vi "Create_Pos_array.vi"(2 "Traverse line":T1 {"Carrier_2 Q (l/min)" format="%#.2f"; "Row Duration (mins)" format="%#.1f"; "Row No" min=0; "Trace Gas Concentration (%)" min=0.0 format="%#_4f"; "Carrier_1 Q (l/min)" format="%#.4f"; "Start X" format="%#.2f"; "Start Y" format="%#.2f"; "Start Z" format="%#.2f"; "End X" format="%#.2f"; "End Y" format="%#.2f"; "End Z" format="%#.2f"; "Tunnel Speed" format="%#.2f"; "Averaging time (mins)" min=0.0 format="%#.2f"}) -> (5 "Traverse line Out":T1 {"Carrier_2 Q (l/min)" format="%#.2f"; "Row Duration (mins)" format="%#.1f"; "Row No" min=0; "Trace Gas Concentration (%)" min=0.0 format="%#_4f"; "Carrier_1 Q (l/min)" format="%#.4f"; "Start X" format="%#.2f"; "Start Y" format="%#.2f"; "Start Z" format="%#.2f"; "End X" format="%#.2f"; "End Y" format="%#.2f"; "End Z" format="%#.2f"; "Tunnel Speed" format="%#.2f"; "Averaging time (mins)" min=0.0 format="%#.2f"}, 6 "Error Messages":string, 7 "Array of Positions":sgl[][](array[numeric]) format="%.2f", 9 "Axis Traversed":enum16{"X traverse", "Y traverse", "Z traverse"}(ring))   [LabVIEW 2020]
uses:
  Traverse_cluster.ctl
  Spacing.ctl
  Controls/Multi_run_mode.ctl
  Globals/Extra_Commands_Global.vi
panel:
  # "X           Y          Z"
  # "Start"
  # "End"
  # "X           Y          Z"
  # "Start"
  # "End"
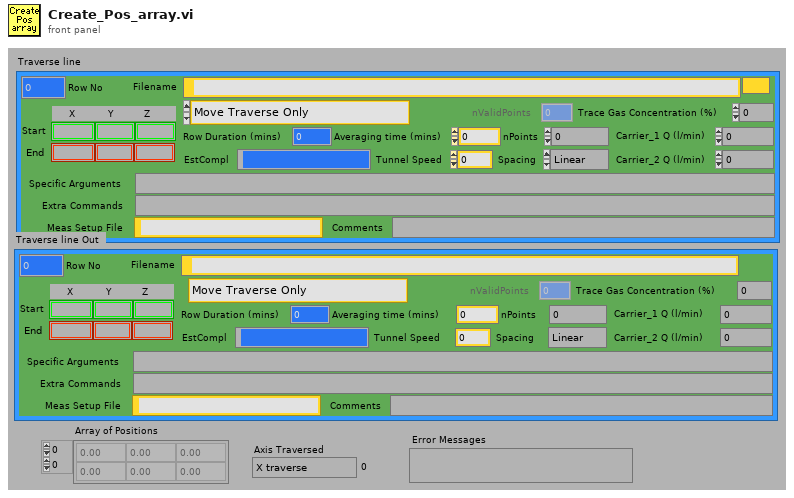
[diagram p1: front panel]
types:
  T1 = typedef "Traverse_cluster.ctl" = cluster{"Start X":sgl, "Start Y":sgl, "Start Z":sgl, "End X":sgl, "End Y":sgl, "End Z":sgl, "nPoints":i32, "Spacing":T2, "Filename":path, "Tunnel Speed":dbl, "Averaging time (mins)":dbl, "Extra Commands":string, "Carrier_1 Q (l/min)":dbl, "Carrier_2 Q (l/min)":dbl, "Trace Gas Concentration (%)":dbl, "Specific Arguments":string, "Comments":string, "Row No":i32, "Row Type Selector":T3, "EstCompl":string, "Row Duration (mins)":dbl, "nValidPoints":i32, "Meas Setup File":string}
  T2 = typedef "Spacing.ctl" = enum16{"Linear", "Log", "Gauss", "Specified", "N/A"}
  T3 = typedef "Multi_run_mode.ctl" = enum16{"Move Traverse Only", "Set Tunnel Speed Only", "Set Source Only", "Set Measurement Conditions", "Single Measurement", "Vertical Profile", "Lateral Profile", "Longitudinal Profile", "Multi-Axis Profile", "Explore Volume", "Auto Calibrate", "Meas Fast FID Bkgnd", "Check Beam Power", "Scanning Valve Measurement", "Run VI Named:", "Set ADAM Ch", "Wait (minutes)", "Send Message", "Synchronize With:", "Fall Back to this Row", "Turn Off Row Repeating", "Traverse 3D Volume", "Blank Row", "Jump to Fall Back Row"}
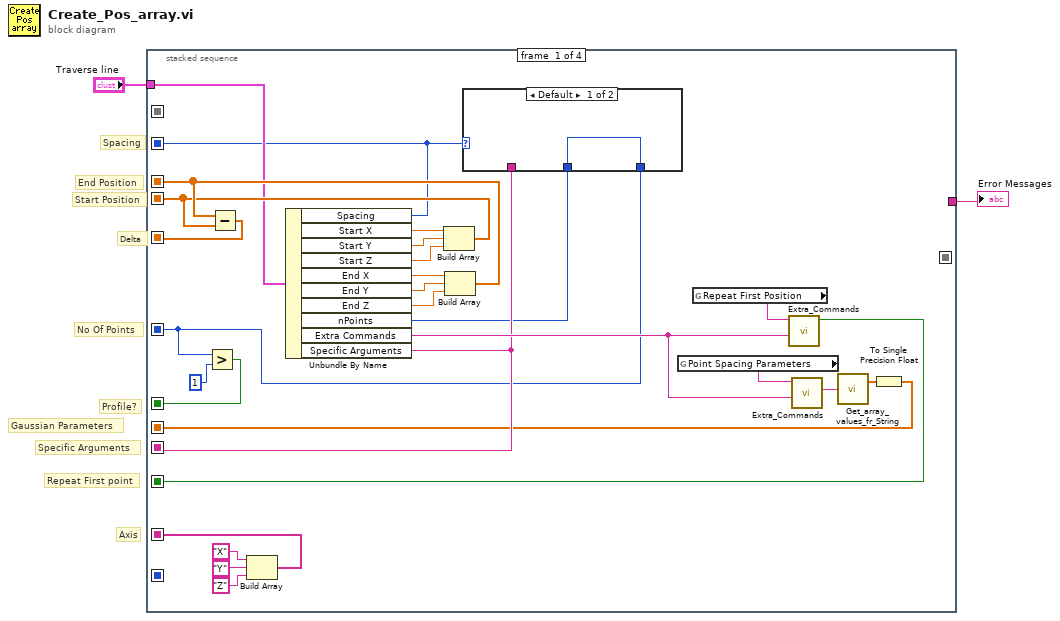
[diagram p0: block diagram]
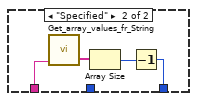
[diagram p2: hidden frame]
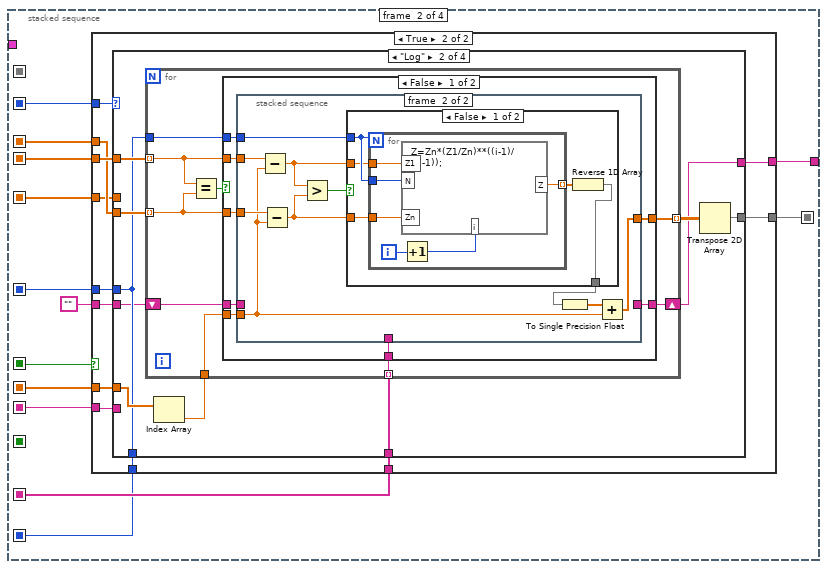
[diagram p3: hidden frame]
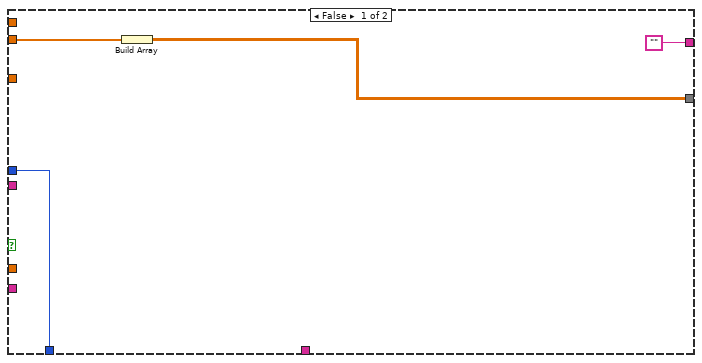
[diagram p4: hidden frame]
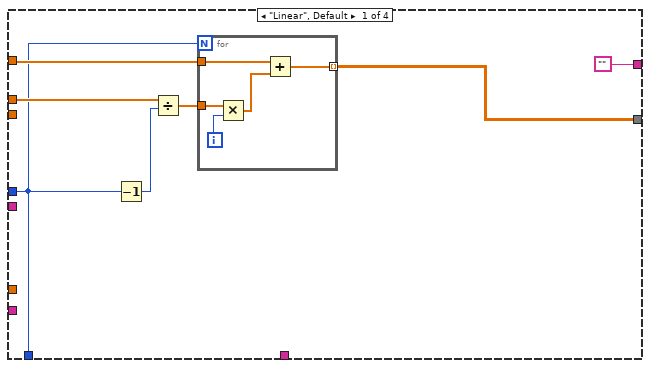
[diagram p5: hidden frame]
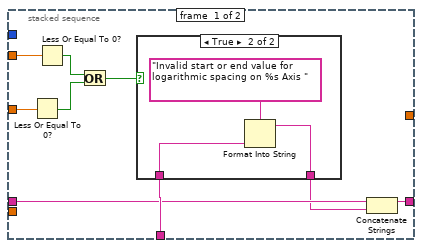
[diagram p6: hidden frame]
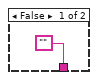
[diagram p7: hidden frame]
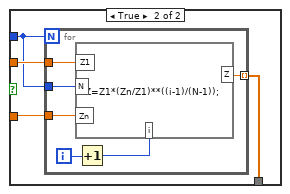
[diagram p8: hidden frame]
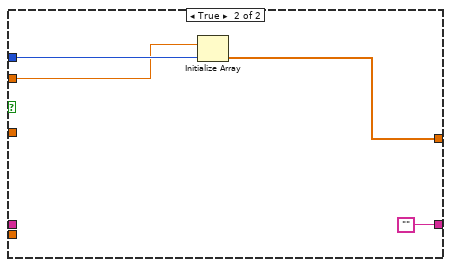
[diagram p9: hidden frame]
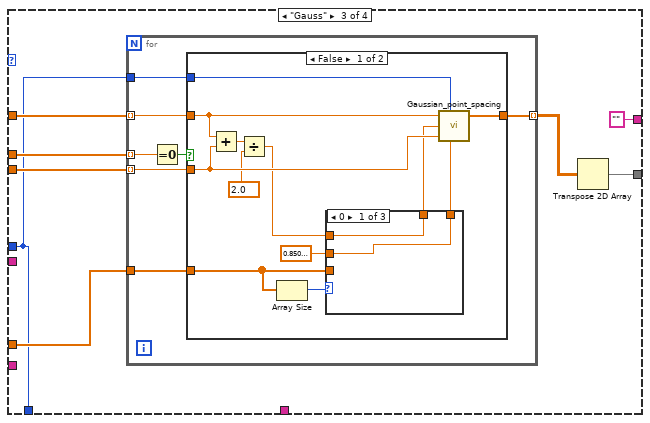
[diagram p10: hidden frame]
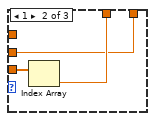
[diagram p11: hidden frame]
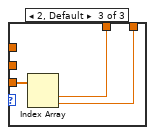
[diagram p12: hidden frame]
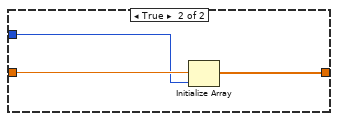
[diagram p13: hidden frame]
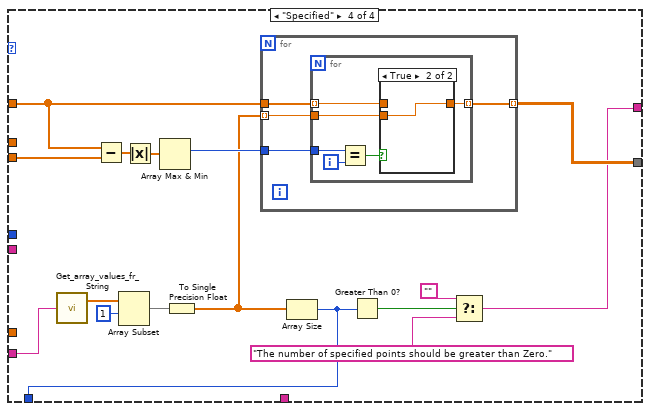
[diagram p14: hidden frame]
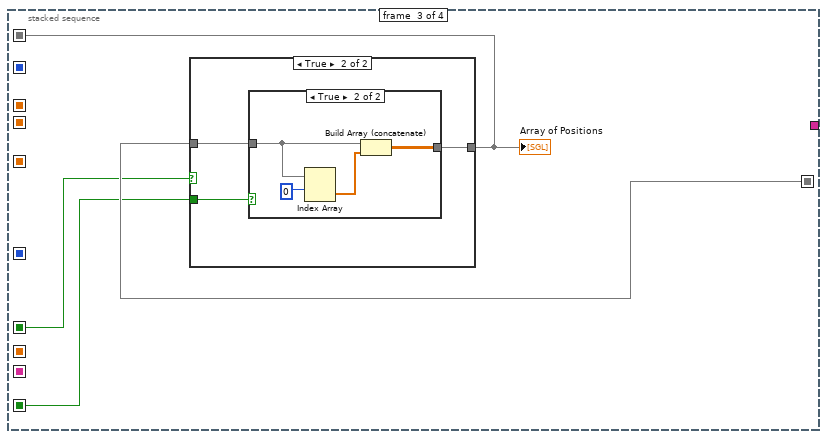
[diagram p16: hidden frame]
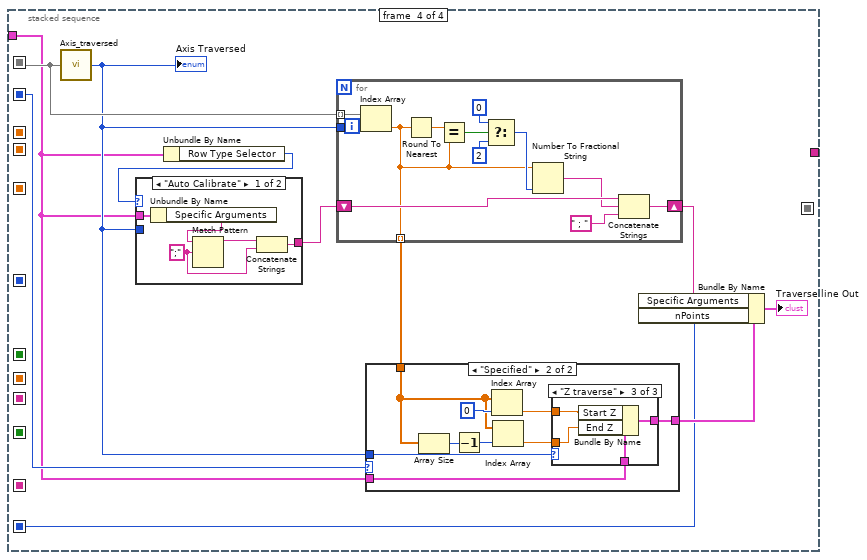
[diagram p19: hidden frame]
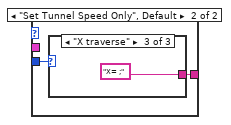
[diagram p20: hidden frame]
diagram:
  # "Gaussian Parameters"
  # "Axis"
  # "Profile?"
  # "Delta"
  # "Repeat First point"
  # "Spacing"
  # "No Of Points"
  # "Specific Arguments"
  # "End Position"
  # "Start Position"
  n1 = stacked-sequence {
    seq-local: [_ w47 _ _] -> [_ _ w220 _]
    seq-local: [w19 _ _ _] -> [_ w44 _ _]
    seq-local: [w22 _ _ _] -> [_ w42 _ _]
    seq-local: [w23 _ _ _] -> [_ w43 _ _]
    seq-local: [w6 _ _ _] -> [_ w40 _ _]
    seq-local: [w7 _ _ _] -> [_ w46 _ _]
    seq-local: [w8 _ _ _] -> [_ w45 _ w236]
    seq-local: [w13 _ _ _] -> [_ _ w219 _]
    seq-local: [w20 _ _ _] -> [_ w39 w218 _]
    seq-local: [w15 _ _ _] -> [_ w38 _ _]
    seq-local: [_ _ w217 _] -> [_ _ _ w240]
    seq-local: [w3 _ _ _] -> [_ w37 _ _]
    seq-local: [_ w36 _ _] -> [_ _ _ w230]
    tunnel: [_ w41 _ _] -> w2
    tunnel: "Traverse line" -> [w12 _ _ w231]
    frame #0 {
      n2 = Build Array("X", "Y", "Z") -> (w15:string[])
      n3 = Unbundle By Name(w12) -> ("Spacing"=w8:T2, "Start X"=w29:sgl, "Start Y"=w28:sgl, "Start Z"=w27:sgl, "End X"=w26:sgl, "End Y"=w25:sgl, "End Z"=w24:sgl, "nPoints"=w5:i32, "Extra Commands"=w10:string, "Specific Arguments"=w7:string)
      n4 = Build Array(w29, w28, w27) -> (w19:sgl[])
      n5 = Build Array(w26, w25, w24) -> (w23:sgl[])
      n6 = Subtract(x=w23, y=w19) -> (x-y=w22:sgl[])
      n7 = case shown="Default" w8 {
        tunnel: w7 -> [_ w34]
        tunnel: [w30 w31] -> w6
        tunnel: w5 -> [w30 _]
        frame Default {
        }
        frame "Specified" {
          n8 = call "Get_array_values_fr_String.vi"("String Value"=w34) -> ("String array"=w33:string[])  [unwired: 1 out]
          n9 = Array Size(array=w33) -> (size(s)=w32:i32)
          n10 = Decrement(x=w32) -> (x-1=w31:i32)
        }
      }
      n11 = Greater?(x=w6, y=1) -> (0:w20:bool)
      n12 = global read "Extra_Commands_Global.vi" "Point Spacing Parameters"() -> (w11:string)
      n13 = global read "Extra_Commands_Global.vi" "Repeat First Position"() -> (w14:string)
      n14 = call "Extra_Commands.vi"("String to Search"=w10, "Command"=w14) -> ("Command Found"=w13:bool)  [unwired: 1 in, 4 out]
      n15 = call "Extra_Commands.vi"("String to Search"=w10, "Command"=w11) -> ("String Value"=w9:string)  [unwired: 1 in, 4 out]
      n16 = call "Get_array_values_fr_String.vi"("String Value"=w9) -> ("Numeric Array"=w4:dbl[])  [unwired: 1 out]
      n17 = To Single Precision Float(number=w4) -> (single precision float=w3:sgl[])
    }
    frame #1 {
      n18 = case shown="True" w39 {
        tunnel: [w50 w63] -> w47
        tunnel: w46 -> [_ w62]
        tunnel: w45 -> [_ w61]
        tunnel: w44 -> [w51 w60]
        tunnel: w43 -> [_ w59]
        tunnel: w42 -> [_ w58]
        tunnel: w40 -> [w48 w57]
        tunnel: ["" w56] -> w41
        tunnel: w38 -> [_ w55]
        tunnel: w37 -> [_ w54]
        tunnel: [w48 w53] -> w36
        tunnel: "" -> [_ w52]
        frame False {
          n19 = Build Array(w51) -> (w50:sgl[][])
        }
        frame True {
          n20 = case shown="\"Log\"" w61 {
            tunnel: w59 -> [_ w84 w156 w199]
            tunnel: w60 -> [w69 w85 w157 w195]
            tunnel: w57 -> [w64 w77 w151 _]
            tunnel: [w70 w83 w155 w203] -> w63
            tunnel: w58 -> [w68 _ w158 _]
            tunnel: w62 -> [_ _ _ w204]
            tunnel: ["" w80 "" ("f") w200] -> w56
            tunnel: w55 -> [_ w81 _ _]
            tunnel: w54 -> [_ w79 w152 _]
            tunnel: [w64 w77 w151 w192] -> w53
            tunnel: w52 -> [_ w76 _ _]
            frame "Linear", Default {
              n21 = Decrement(x=w64) -> (x-1=w66:i32)
              n22 = Divide(x=w68, y=w66) -> (x/y=w67:sgl[])
              n23 = for {
                N: w64 -> [_]
                tunnel: w67 -> [w74]
                tunnel: w69 -> [w72]
                tunnel: [w71] -> w70 mode=indexing
                i -> [w75]
                n24 = Multiply(x=w74, y=w75) -> (x*y=w73:sgl[])
                n25 = Add(x=w72, y=w73) -> (x+y=w71:sgl[])
              }
            }
            frame "Log" {
              n26 = Index Array(array=w79) -> (element=w78:sgl)  [unwired: 1 in]
              n27 = for {
                tunnel: [w94] -> w82 mode=indexing
                tunnel: w85 -> [w87] mode=indexing
                tunnel: w84 -> [w86] mode=indexing
                tunnel: w77 -> [w93]
                tunnel: w81 -> [w91] mode=indexing
                shift-right: [w89] -> w80
                shift-left: w76 -> [w90]
                tunnel: w78 -> [w88]
                n28 = Equal?(x=w87, y=w86) -> (x = y?=w92:bool)
                n29 = case shown="False" w92 {
                  tunnel: w93 -> [w102 w149]
                  tunnel: w86 -> [w101 _]
                  tunnel: w87 -> [w100 w148]
                  tunnel: [w99 w150] -> w94
                  tunnel: w91 -> [w98 _]
                  tunnel: w90 -> [w97 _]
                  tunnel: [w96 ""] -> w89
                  tunnel: w88 -> [w95 _]
                  frame False {
                    n30 = stacked-sequence {
                      tunnel: [_ w123] -> w99
                      tunnel: w100 -> [w111 w122]
                      tunnel: w101 -> [w110 w121]
                      tunnel: w102 -> [_ w124]
                      tunnel: w98 -> [w106 _]
                      tunnel: w97 -> [w105 _]
                      tunnel: [w103 _] -> w96
                      tunnel: w95 -> [_ w120]
                      frame #0 {
                        n31 = Less Or Equal To 0?(x=w110) -> (x <= 0?=w109:bool)
                        n32 = Less Or Equal To 0?(x=w111) -> (x <= 0?=w108:bool)
                        n33 = Or(x=w108, y=w109) -> (x .or. y?=w107:bool)
                        n34 = case shown="True" w107 {
                          tunnel: w106 -> [_ w115]
                          tunnel: ["" w113] -> w104
                          frame False {
                          }
                          frame True {
                            n35 = Format Into String(format string="Invalid start or end value for logarithmic spacing on %s Axis " ("Format String"), w115) -> (resulting string=w113:string)  [unwired: 2 in, 1 out]
                          }
                        }
                        n36 = Concatenate Strings(w105, w104) -> (w103:string)
                      }
                      frame #1 {
                        n37 = Subtract(x=w122, y=w120) -> (x-y=w118:sgl)
                        n38 = Subtract(x=w121, y=w120) -> (x-y=w119:sgl)
                        n39 = Greater?(x=w118, y=w119) -> (0:w125:bool)
                        n40 = case shown="False" w125 {
                          tunnel: [w127 w137] -> w117
                          tunnel: w118 -> [w126 w140]
                          tunnel: w119 -> [w130 w139]
                          tunnel: w124 -> [w129 w138]
                          frame False {
                            n41 = for {
                              N: w129 -> [_]
                              tunnel: w130 -> [w133]
                              tunnel: w129 -> [w132]
                              tunnel: [w134] -> w128 mode=indexing
                              tunnel: w126 -> [w131]
                              i -> [w136]
                              n42 = Increment(x=w136) -> (x+1=w135:i32)
                              n43 = formula code="Z=Zn*(Z1/Zn)**((i-1)/(N-1));"("i"=w135, "N"=w132, "Zn"=w133, "Z1"=w131) -> ("Z"=w134:dbl)
                            }
                            n44 = Reverse 1D Array(array=w128) -> (reversed array=w127:dbl[])
                          }
                          frame True {
                            n45 = for {
                              N: w138 -> [_]
                              tunnel: w140 -> [w146]
                              tunnel: w139 -> [w145]
                              tunnel: w138 -> [w142]
                              tunnel: [w141] -> w137 mode=indexing
                              i -> [w144]
                              n46 = Increment(x=w144) -> (x+1=w143:i32)
                              n47 = formula code="Z=Z1*(Zn/Z1)**((i-1)/(N-1));"("i"=w143, "N"=w142, "Zn"=w145, "Z1"=w146) -> ("Z"=w141:dbl)
                            }
                          }
                        }
                        n48 = To Single Precision Float(number=w117) -> (single precision float=w116:sgl[])
                        n49 = Add(x=w116, y=w120) -> (x+y=w123:sgl[])
                      }
                    }
                  }
                  frame True {
                    n50 = Initialize Array(w148, w149) -> (w150:sgl[])
                  }
                }
              }
              n51 = Transpose 2D Array(2D array=w82) -> (transposed array=w83:sgl[][])
            }
            frame "Gauss" {
              n52 = for {
                tunnel: w158 -> [w160] mode=indexing
                tunnel: w157 -> [w164] mode=indexing
                tunnel: w156 -> [w163] mode=indexing
                tunnel: w151 -> [w162]
                tunnel: [w161] -> w154 mode=indexing
                tunnel: w152 -> [w159]
                n53 = Equal To 0?(x=w160) -> (x = 0?=w165:bool)
                n54 = case shown="False" w165 {
                  tunnel: w164 -> [w175 w188]
                  tunnel: w163 -> [w174 _]
                  tunnel: w162 -> [w177 w187]
                  tunnel: [w176 w186] -> w161
                  tunnel: w159 -> [w167 _]
                  frame False {
                    n55 = Add(x=w175, y=w174) -> (x+y=w173:sgl)
                    n56 = Divide(x=w173, y=sgl 2.0) -> (x/y=w169:sgl)
                    n57 = Array Size(array=w167) -> (size(s)=w171:i32)
                    n58 = case shown="0" w171 {
                      tunnel: [w179 w181 w184] -> w170
                      tunnel: w169 -> [w179 _ _]
                      tunnel: [w178 w180 w183] -> w168
                      tunnel: w167 -> [_ w182 w185]
                      tunnel: sgl 0.85 ("Guass intensity") -> [w178 w180 _]
                      frame 0 {
                      }
                      frame 1 {
                        n59 = Index Array(array=w182) -> (element=w181:sgl)  [unwired: 1 in]
                      }
                      frame 2, Default {
                        n60 = Index Array(array=w185) -> (element #1=w184:sgl, element #2=w183:sgl)  [unwired: 2 in]
                      }
                    }
                    n61 = call "Gaussian_point_spacing.vi"("Start point"=w175, "No of points"=w177, "Centre point"=w170, "End point"=w174, "Guass intensity"=w168) -> ("Positions"=w176:sgl[])  [unwired: 2 out]
                  }
                  frame True {
                    n62 = Initialize Array(w188, w187) -> (w186:sgl[])
                  }
                }
              }
              n63 = Transpose 2D Array(2D array=w154) -> (transposed array=w155:sgl[][])
            }
            frame "Specified" {
              n64 = call "Get_array_values_fr_String.vi"("String Value"=w204) -> ("Numeric Array"=w194:dbl[])  [unwired: 1 out]
              n65 = Subtract(x=w195, y=w199) -> (x-y=w198:sgl[])
              n66 = Array Subset(array=w194, index=1) -> (w190:dbl[])  [unwired: 1 in]
              n67 = Absolute Value(x=w198) -> (abs(x)=w197:sgl[])
              n68 = Array Max & Min(array=w197) -> (max index (indices)=w196:i32)  [unwired: 3 out]
              n69 = To Single Precision Float(number=w190) -> (single precision float=w189:sgl[])
              n70 = for {
                tunnel: w189 -> [w206] mode=indexing
                tunnel: [w207] -> w203 mode=indexing
                tunnel: w196 -> [w208]
                tunnel: w195 -> [w205]
                n71 = for {
                  tunnel: w208 -> [w212]
                  tunnel: [w214] -> w207 mode=indexing
                  tunnel: w206 -> [w213]
                  tunnel: w205 -> [w209] mode=indexing
                  i -> [w211]
                  n72 = Equal?(x=w212, y=w211) -> (x = y?=w210:bool)
                  n73 = case shown="True" w210 {
                    tunnel: [w215 w216] -> w214
                    tunnel: w213 -> [_ w216]
                    tunnel: w209 -> [w215 _]
                    frame False {
                    }
                    frame True {
                    }
                  }
                }
              }
              n74 = Array Size(array=w189) -> (size(s)=w192:i32)
              n75 = Greater Than 0?(x=w192) -> (x > 0?=w191:bool)
              n76 = Select(t="", s=w191, f="The number of specified points should be greater than Zero.") -> (s? t:f=w200:string)
            }
          }
        }
      }
    }
    frame #2 {
      n77 = case shown="True" w218 {
        tunnel: [w221 w224] -> w217
        tunnel: w220 -> [w221 w223]
        tunnel: w219 -> [_ w222]
        frame False {
        }
        frame True {
          n78 = case shown="True" w222 {
            tunnel: [w225 w229] -> w224
            tunnel: w223 -> [w225 w227]
            frame False {
            }
            frame True {
              n79 = Index Array(array=w227, index (row)=0) -> (element=w228:sgl[])  [unwired: 1 in]
              n80 = Build Array (concatenate)(w227, w228) -> (w229:sgl[][])
            }
          }
        }
      }
      "Array of Positions" <- w217
    }
    frame #3 {
      n81 = call "Axis_traversed.vi"("Position array"=w240) -> ("Axis Traversed"=w234:enum16{"X traverse", "Y traverse", "Z traverse"})  [unwired: 4 out]
      "Axis Traversed" <- w234
      n82 = Unbundle By Name(w231) -> ("Row Type Selector"=w232:T3)
      n83 = case shown="\"Auto Calibrate\"" w232 {
        tunnel: [w243 w247] -> w237
        tunnel: w234 -> [_ w246]
        tunnel: w231 -> [w245 _]
        frame "Auto Calibrate" {
          w241 = ";" ("regular expression")
          n84 = Unbundle By Name(w245) -> ("Specific Arguments"=w244:string)
          n85 = Match Pattern(string=w244, regular expression=w241) -> (before substring=w242:string)  [unwired: 4 out]
          n86 = Concatenate Strings(w242, w241) -> (w243:string)
        }
        frame "Set Tunnel Speed Only", Default {
          n87 = case shown="\"X traverse\"" w246 {
            tunnel: ["Y= ;" "Z= ;" "X= ;"] -> w247
            frame "Y traverse" {
            }
            frame "Z traverse" {
            }
            frame "X traverse" {
            }
          }
        }
      }
      n88 = for {
        tunnel: w234 -> [w284]
        tunnel: w240 -> [w274] mode=indexing
        shift-right: [w282] -> w239
        shift-left: w237 -> [w283]
        tunnel: [w273] -> w235 mode=indexing
        n89 = Index Array(array=w274, index=w284) -> (element=w273:sgl)
        n90 = Round To Nearest(number=w273) -> (nearest integer value=w276:sgl)
        n91 = Equal?(x=w276, y=w273) -> (x = y?=w275:bool)
        n92 = Select(t=0, s=w275, f=2) -> (s? t:f=w279:i32)
        n93 = Number To Fractional String(number=w273, precision (6)=w279) -> (F-format string=w281:string)  [unwired: 2 out]
        n94 = Concatenate Strings(w283, w281, " ; " ("string")) -> (w282:string)
      }
      n95 = case shown="\"Specified\"" w236 {
        tunnel: w235 -> [_ w255]
        tunnel: w234 -> [_ w260]
        tunnel: w231 -> [w251 w259]
        tunnel: [w251 w254] -> w233
        frame "Linear", Default {
        }
        frame "Specified" {
          n96 = Array Size(array=w255) -> (size(s)=w258:i32)
          n97 = Decrement(x=w258) -> (x-1=w256:i32)
          n98 = Index Array(array=w255, index=0) -> (element=w253:sgl)
          n99 = Index Array(array=w255, index=w256) -> (element=w252:sgl)
          n100 = case shown="\"Z traverse\"" w260 {
            tunnel: w259 -> [w264 w268 w272]
            tunnel: [w263 w267 w271] -> w254
            tunnel: w253 -> [w262 w266 w270]
            tunnel: w252 -> [w261 w265 w269]
            frame "X traverse" {
              n101 = Bundle By Name(cluster=w264, "Start X"=w262, "End X"=w261) -> (w263:T1)
            }
            frame "Y traverse" {
              n102 = Bundle By Name(cluster=w268, "Start Y"=w266, "End Y"=w265) -> (w267:T1)
            }
            frame "Z traverse" {
              n103 = Bundle By Name(cluster=w272, "Start Z"=w270, "End Z"=w269) -> (w271:T1)
            }
          }
        }
      }
      n104 = Bundle By Name(cluster=w233, "Specific Arguments"=w239, "nPoints"=w230) -> (→"Traverse line Out":T1)
    }
  }
  "Error Messages" <- w2
